vi "4-libssh2_sftp_read-binary data truncated.vi"() -> ()   [LabVIEW 2017, in "bug_reports.lvlib"]
uses:
  bug_reports.lvlib
  libssh2/libssh2.lvlib
  support/support.lvlib
  <vilib>/PNR/Transparent Assertions/Transparent Assertions/Transparent Assertions.lvlib
panel:
  out "error out":errorcluster
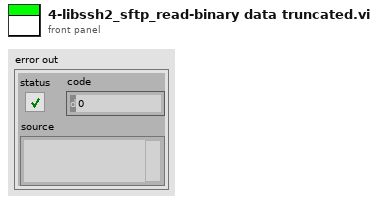
[diagram p1: front panel]
types:
  T1 = typedef "libssh2.lvlib/Session Refnum.ctl" = refnum<k1>
  T2 = typedef "libssh2.lvlib/SFTP Refnum.ctl" = refnum<k1>
  T3 = typedef "libssh2.lvlib/SFTP Handle Refnum.ctl" = refnum<k1>
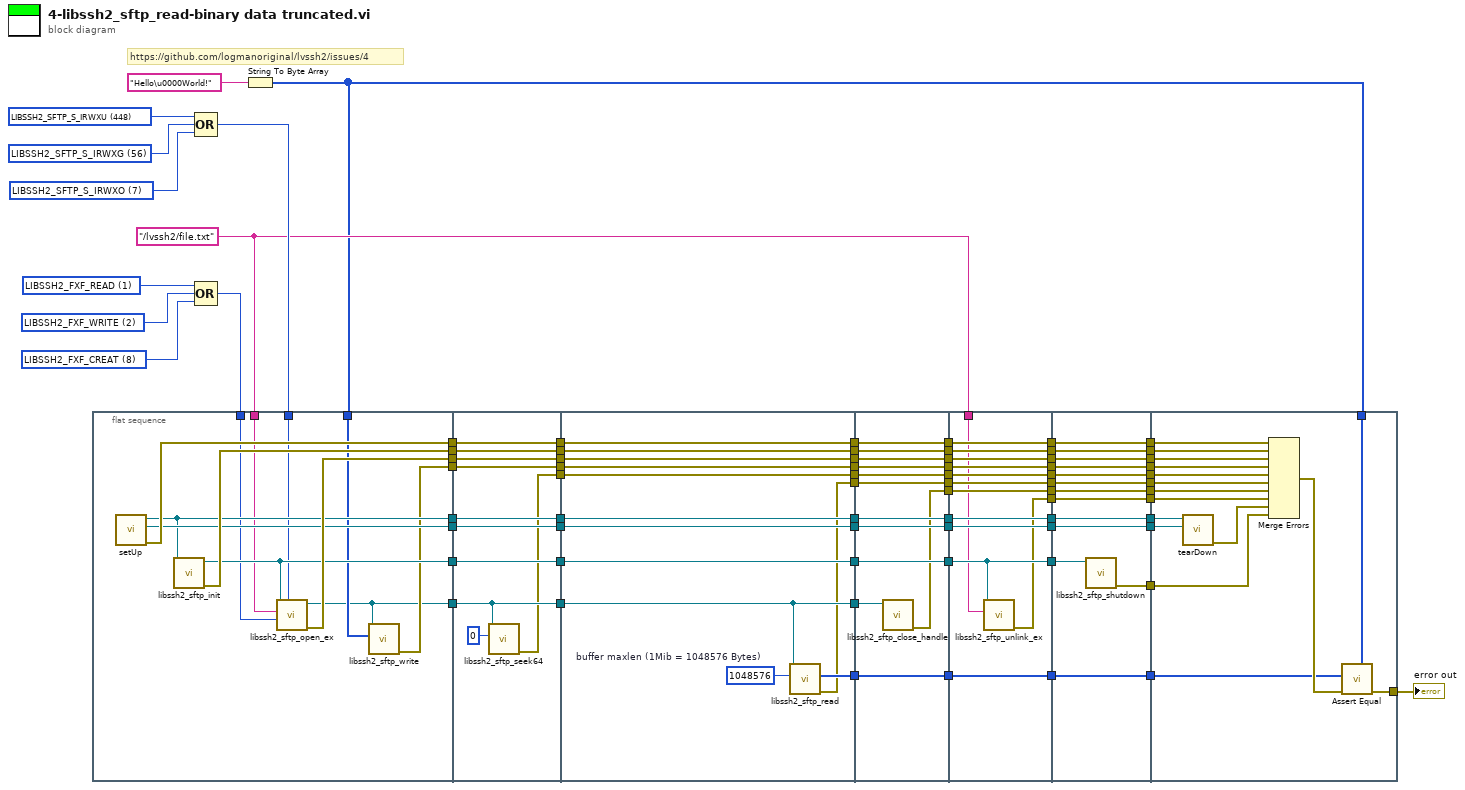
[diagram p0: block diagram]
diagram:
  w6 = u32 2 items=["LIBSSH2_FXF_READ"=1, "LIBSSH2_FXF_WRITE"=2, "LIBSSH2_FXF_APPEND"=4, "LIBSSH2_FXF_CREAT"=8, "LIBSSH2_FXF_TRUNC"=16, "LIBSSH2_FXF_EXCL"=32] ("flags")
  w7 = u32 1 items=["LIBSSH2_FXF_READ"=1, "LIBSSH2_FXF_WRITE"=2, "LIBSSH2_FXF_APPEND"=4, "LIBSSH2_FXF_CREAT"=8, "LIBSSH2_FXF_TRUNC"=16, "LIBSSH2_FXF_EXCL"=32] ("flags")
  w5 = u32 8 items=["LIBSSH2_FXF_READ"=1, "LIBSSH2_FXF_WRITE"=2, "LIBSSH2_FXF_APPEND"=4, "LIBSSH2_FXF_CREAT"=8, "LIBSSH2_FXF_TRUNC"=16, "LIBSSH2_FXF_EXCL"=32] ("flags")
  w2 = "/lvssh2/file.txt" ("filename")
  w9 = 7 items=["LIBSSH2_SFTP_S_IRWXU"=448, "LIBSSH2_SFTP_S_IRUSR"=256, "LIBSSH2_SFTP_S_IWUSR"=128, "LIBSSH2_SFTP_S_IXUSR"=64, "LIBSSH2_SFTP_S_IRWXG"=56, "LIBSSH2_SFTP_S_IRGRP"=32, "LIBSSH2_SFTP_S_IWGRP"=16, "LIBSSH2_SFTP_S_IXGRP"=8, "LIBSSH2_SFTP_S_IRWXO"=7, "LIBSSH2_SFTP_S_IROTH"=4, "LIBSSH2_SFTP_S_IWOTH"=2, "LIBSSH2_SFTP_S_IXOTH"=1] ("mode")
  w10 = 56 items=["LIBSSH2_SFTP_S_IRWXU"=448, "LIBSSH2_SFTP_S_IRUSR"=256, "LIBSSH2_SFTP_S_IWUSR"=128, "LIBSSH2_SFTP_S_IXUSR"=64, "LIBSSH2_SFTP_S_IRWXG"=56, "LIBSSH2_SFTP_S_IRGRP"=32, "LIBSSH2_SFTP_S_IWGRP"=16, "LIBSSH2_SFTP_S_IXGRP"=8, "LIBSSH2_SFTP_S_IRWXO"=7, "LIBSSH2_SFTP_S_IROTH"=4, "LIBSSH2_SFTP_S_IWOTH"=2, "LIBSSH2_SFTP_S_IXOTH"=1] ("mode")
  w11 = 448 items=["LIBSSH2_SFTP_S_IRWXU"=448, "LIBSSH2_SFTP_S_IRUSR"=256, "LIBSSH2_SFTP_S_IWUSR"=128, "LIBSSH2_SFTP_S_IXUSR"=64, "LIBSSH2_SFTP_S_IRWXG"=56, "LIBSSH2_SFTP_S_IRGRP"=32, "LIBSSH2_SFTP_S_IWGRP"=16, "LIBSSH2_SFTP_S_IXGRP"=8, "LIBSSH2_SFTP_S_IRWXO"=7, "LIBSSH2_SFTP_S_IROTH"=4, "LIBSSH2_SFTP_S_IWOTH"=2, "LIBSSH2_SFTP_S_IXOTH"=1] ("mode")
  # "https://github.com/logmanoriginal/lvssh2/issues/4"
  n1 = flat-sequence {
    tunnel: [w87] -> w75
    tunnel: [w86] -> w74
    tunnel: [w85] -> w73
    tunnel: [w84] -> w72
    tunnel: [w83] -> w71
    tunnel: [w82] -> w70
    tunnel: [w76] -> w69
    tunnel: w1 -> [w81]
    tunnel: [w80] -> w68
    tunnel: w4 -> [w77]
    tunnel: w2 -> [w78]
    tunnel: w8 -> [w79]
    tunnel: w75 -> [w97]
    tunnel: [w97] -> w67
    tunnel: w74 -> [w96]
    tunnel: [w96] -> w66
    tunnel: w73 -> [w95]
    tunnel: [w95] -> w65
    tunnel: w72 -> [w94]
    tunnel: [w94] -> w64
    tunnel: w71 -> [w93]
    tunnel: [w93] -> w63
    tunnel: w70 -> [w92]
    tunnel: [w92] -> w62
    tunnel: w69 -> [w90]
    tunnel: [w90] -> w61
    tunnel: w68 -> [w91]
    tunnel: [w91] -> w60
    tunnel: [w89] -> w59
    tunnel: w67 -> [w109]
    tunnel: [w109] -> w58
    tunnel: w66 -> [w108]
    tunnel: [w108] -> w57
    tunnel: w65 -> [w107]
    tunnel: [w107] -> w56
    tunnel: w64 -> [w106]
    tunnel: [w106] -> w55
    tunnel: w63 -> [w105]
    tunnel: [w105] -> w54
    tunnel: w62 -> [w104]
    tunnel: [w104] -> w53
    tunnel: w61 -> [w101]
    tunnel: [w101] -> w52
    tunnel: w60 -> [w103]
    tunnel: [w103] -> w51
    tunnel: [w100] -> w50
    tunnel: [w99] -> w49
    tunnel: w59 -> [w98]
    tunnel: [w98] -> w48
    tunnel: [w115] -> w41
    tunnel: w58 -> [w121]
    tunnel: [w121] -> w42
    tunnel: w57 -> [w120]
    tunnel: [w120] -> w43
    tunnel: w56 -> [w119]
    tunnel: [w119] -> w44
    tunnel: w55 -> [w118]
    tunnel: [w118] -> w45
    tunnel: w54 -> [w117]
    tunnel: [w117] -> w46
    tunnel: w53 -> [w116]
    tunnel: [w116] -> w47
    tunnel: w52 -> [w114]
    tunnel: w51 -> [w113]
    tunnel: [w113] -> w40
    tunnel: [w112] -> w39
    tunnel: w50 -> [w112]
    tunnel: [w111] -> w38
    tunnel: w49 -> [w111]
    tunnel: w48 -> [w110]
    tunnel: [w110] -> w37
    tunnel: w47 -> [w134]
    tunnel: [w134] -> w36
    tunnel: w46 -> [w133]
    tunnel: [w133] -> w35
    tunnel: w45 -> [w124]
    tunnel: [w124] -> w34
    tunnel: w44 -> [w132]
    tunnel: [w132] -> w33
    tunnel: w43 -> [w131]
    tunnel: [w131] -> w32
    tunnel: w42 -> [w130]
    tunnel: [w130] -> w31
    tunnel: w41 -> [w129]
    tunnel: [w129] -> w30
    tunnel: w40 -> [w128]
    tunnel: [w128] -> w29
    tunnel: w39 -> [w127]
    tunnel: [w127] -> w28
    tunnel: w38 -> [w126]
    tunnel: [w126] -> w27
    tunnel: w37 -> [w125]
    tunnel: [w125] -> w26
    tunnel: w2 -> [w123]
    tunnel: [w122] -> w25
    tunnel: w36 -> [w147]
    tunnel: [w147] -> w24
    tunnel: w35 -> [w146]
    tunnel: [w146] -> w23
    tunnel: w34 -> [w143]
    tunnel: w33 -> [w145]
    tunnel: [w145] -> w22
    tunnel: w32 -> [w144]
    tunnel: [w144] -> w21
    tunnel: [w142] -> w20
    tunnel: w31 -> [w141]
    tunnel: [w141] -> w19
    tunnel: [w140] -> w18
    tunnel: w30 -> [w140]
    tunnel: w29 -> [w139]
    tunnel: [w139] -> w17
    tunnel: [w138] -> w16
    tunnel: w28 -> [w138]
    tunnel: [w137] -> w15
    tunnel: w27 -> [w137]
    tunnel: w26 -> [w136]
    tunnel: [w136] -> w14
    tunnel: w25 -> [w135]
    tunnel: [w135] -> w13
    tunnel: w24 -> [w163]
    tunnel: w23 -> [w162]
    tunnel: w22 -> [w161]
    tunnel: [w158] -> w12
    tunnel: w21 -> [w157]
    tunnel: w20 -> [w156]
    tunnel: w19 -> [w155]
    tunnel: w18 -> [w154]
    tunnel: w17 -> [w153]
    tunnel: w16 -> [w152]
    tunnel: w15 -> [w151]
    tunnel: w1 -> [w150]
    tunnel: w14 -> [w149]
    tunnel: w13 -> [w148]
    frame #0 {
      n2 = call "setUp.vi"() -> ("error out"=w85:errorcluster, "connection ID"=w83:refnum<k5>, "session"=w82:T1)  [unwired: 9 in]
      n3 = call "libssh2_sftp_init.vi"("session"=w82) -> ("error out"=w86:errorcluster, "sftp"=w84:T2)  [unwired: 9 in]
      n4 = call "libssh2_sftp_open_ex.vi"("mode"=w79, "flags"=w77, "filename"=w78, "sftp"=w84) -> ("error out"=w87:errorcluster, "sftp handle"=w76:T3)  [unwired: 6 in]
      n5 = call "libssh2_sftp_write.vi"("buffer"=w81, "sftp handle"=w76) -> ("error out"=w80:errorcluster)  [unwired: 8 in, 1 out]
    }
    frame #1 {
      n6 = call "libssh2_sftp_seek64.vi"("offset"=u64 0, "sftp handle"=w90) -> ("error out"=w89:errorcluster)  [unwired: 9 in]
    }
    frame #2 {
      w102 = 1048576  # buffer maxlen (1Mib = 1048576 Bytes)
      n7 = call "libssh2_sftp_read.vi"("buffer maxlen"=w102, "sftp handle"=w101) -> ("error out"=w99:errorcluster, "buffer"=w100:u8[])  [unwired: 7 in, 1 out]
    }
    frame #3 {
      n8 = call "libssh2_sftp_close_handle.vi"("sftp handle"=w114) -> ("error out"=w115:errorcluster)  [unwired: 10 in]
    }
    frame #4 {
      n9 = call "libssh2_sftp_unlink_ex.vi"("file"=w123, "sftp"=w124) -> ("error out"=w122:errorcluster)  [unwired: 9 in]
    }
    frame #5 {
      n10 = call "libssh2_sftp_shutdown.vi"("sftp"=w143) -> ("error out"=w142:errorcluster)  [unwired: 10 in]
    }
    frame #6 {
      n11 = call "tearDown.vi"("connection ID"=w162, "session"=w163) -> ("error out"=w160:errorcluster)  [unwired: 9 in]
      n12 = Merge Errors(w161, w157, w155, w153, w149, w151, w154, w148, w160, w156) -> (w159:errorcluster)
      n13 = call <vilib>:"Assert Equal.vi"("Expected"=w150, "error in (no error)"=w159, "Actual"=w152) -> ("error out"=w158:errorcluster)  [unwired: 8 in]
    }
  }
  n14 = Compound Arithmetic op=OR(w11, w10, w9) -> (w8:i32)
  n15 = Compound Arithmetic op=OR(w7, w6, w5) -> (w4:u32)
  n16 = String To Byte Array(string="Hello\u0000World!" ("buffer")) -> (unsigned byte array=w1:u8[])
  "error out" <- w12
